vi "DestroyPrivateEvents.vi"(8 "error in (no error)":errorcluster, 11 "SMO.UI":refnum<class "SMO.UI.lvclass">) -> (0 "error out":errorcluster, 3 "SMO.UI out":refnum<class "SMO.UI.lvclass">)   [LabVIEW 2021, in "smo.lvlib" / "SMO.UI.lvclass"]
uses:
  SMO.UI.lvclass
  SMO.UI.lvclass/SMO.UI.ctl
  SMO.UI.ReftoDVR.vi
  SMO/SMO.lvclass
panel:
  # "For instructions on how to use the JKI State Machine Objects, examples and video tutorials, visit:\nhttp://jki.net/state-machine-objects/\n\nJKI State Machine Objects™\nhttp://jki.net/state-machine-objects/\nCopyright (C) 2005-2015, JKI <info@jki.net>\nALL RIGHTS RESERVED"
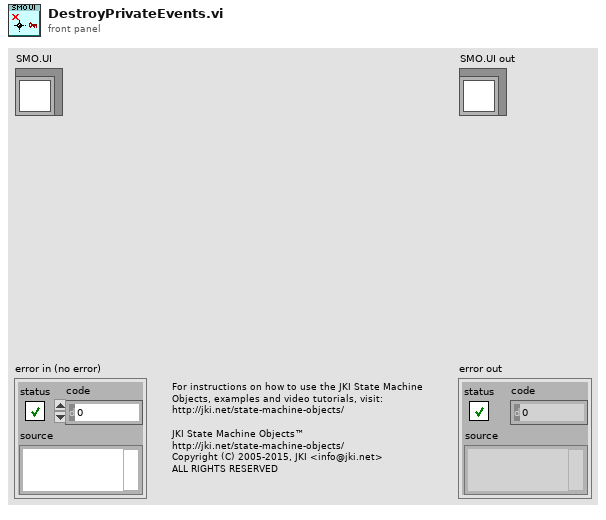
[diagram p1: front panel]
types:
  T1 = typedef "smo.lvlib/SMO.UI.lvclass/PrivateEvents--Cluster.ctl" = cluster{"Show-Hide UI":refnum<user-event>}
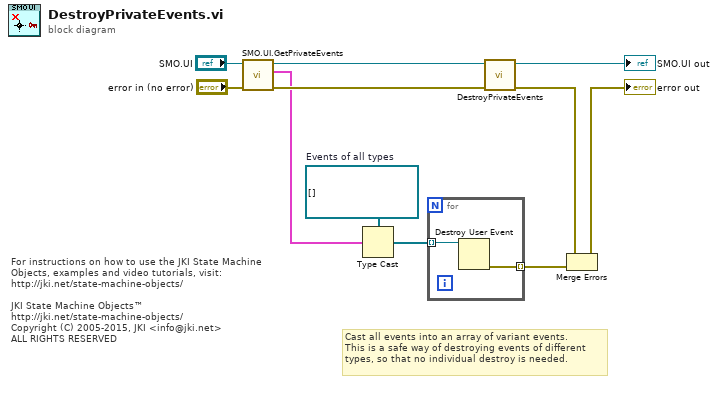
[diagram p0: block diagram]
diagram:
  w4 = refnum<user-event>[] []  # Events of all types
  # "For instructions on how to use the JKI State Machine Objects, examples and video tutorials, visit:\nhttp://jki.net/state-machine-objects/\n\nJKI State Machine Objects™\nhttp://jki.net/state-machine-objects/\nCopyright (C) 2005-2015, JKI <info@jki.net>\nALL RIGHTS RESERVED"
  # "Cast all events into an array of variant events.\nThis is a safe way of destroying events of different\ntypes, so that no individual destroy is needed."
  n1 = call "SMO.UI.GetPrivateEvents.vi"("error in (no error)"="error in (no error)", "SMO.UI"="SMO.UI") -> ("error out"=w9:errorcluster, "SMO.UI Private Events"=w1:T1, "SMO.UI out"=w11:refnum<class "SMO.UI.lvclass">)  [unwired: 7 in]
  n2 = Type Cast(type=w4, x=w1) -> (*(type *) &x=w5:refnum<user-event>[])
  n3 = for {
    tunnel: w5 -> [w13] mode=indexing
    tunnel: [w12] -> w6 mode=indexing
    n4 = Destroy User Event(user event=w13) -> (error out=w12:errorcluster)  [unwired: 1 in]
  }
  n5 = call-parent "DestroyPrivateEvents.vi"("error in (no error)"=w9, "SMO"=w11) -> ("error out"=w3:errorcluster, "SMO out"=→"SMO.UI out":refnum<class "SMO.UI.lvclass">)  [unwired: 8 in]
  n6 = Merge Errors(w3, w6) -> (→"error out":errorcluster)
